vi "Constant - Default TCP Port Number.vi"() -> (3 "Port":u16=9760)   [LabVIEW 2021]
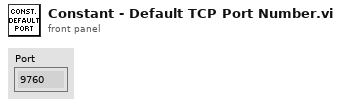
[diagram p1: front panel]
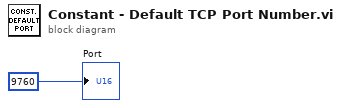
[diagram p0: block diagram]
diagram:
  "Port" <- u16 9760 ("remote port or service name")
